vi "Setup.vi"(0 "Vector 26GHz Path Group in":refnum<class "Vector 26GHz Path Group.lvclass">, 11 "error in":errorcluster) -> (4 "Vector 26GHz Path Group out":refnum<class "Vector 26GHz Path Group.lvclass">, 15 "error out":errorcluster)   [LabVIEW 2023, in "RFFixtureCharact.RMM.lvlib" / "Vector 26GHz Path Group.lvclass"]
uses:
  Vector 26GHz Path Group.lvclass
  Vector 26GHz Path Group.lvclass/Vector 26GHz Path Group.ctl
  Paths/Vector Path/Vector 26GHz Path.lvclass
  Public/Base Classes/Vector/Vector Abstract Path/Vector Abstract Path.lvclass
  Common/RFCalAndFixtureCharact.Common.lvlib
  Public/Base Classes/Vector/Vector Path Group/Vector Path Group.lvclass
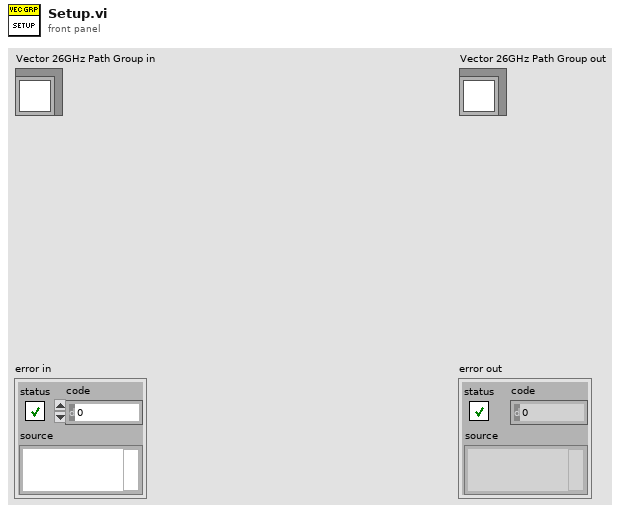
[diagram p1: front panel]
types:
  T1 = typedef "RFFixtureCharact.Public.lvlib/Vector Path Group.lvclass/Sweep.ctl" = cluster{"Port Power":dbl, "Frequencies":dbl[], "Test Receiver Attenuation":dbl, "IF Bandwidth":dbl}
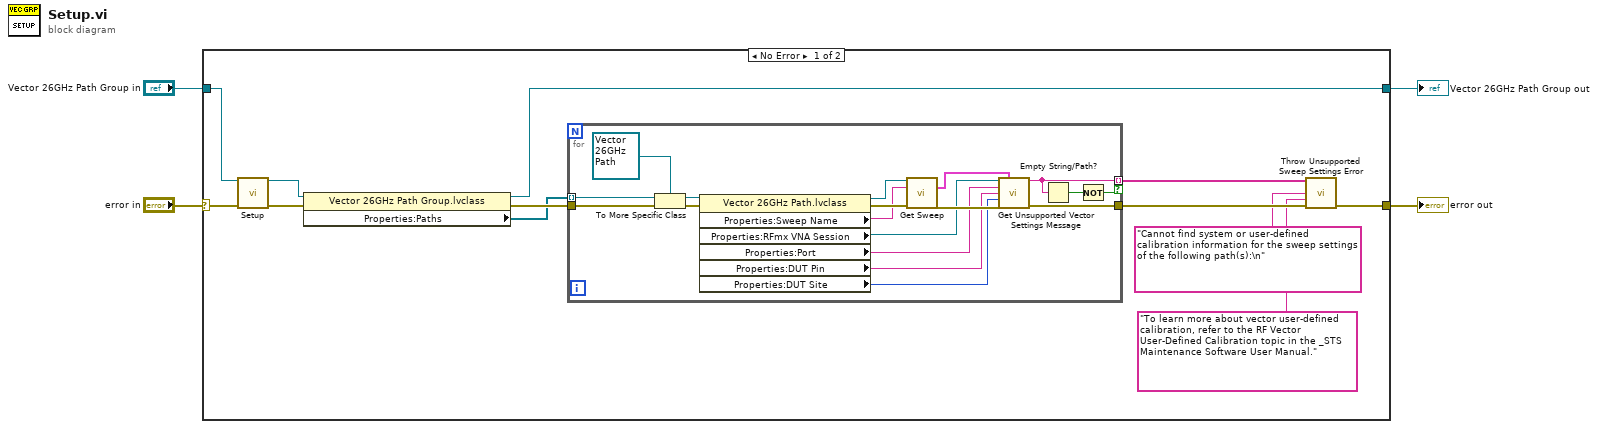
[diagram p0: block diagram]
diagram:
  n1 = case shown="No Error" "error in" {
    selector: "error in" -> [w16 w36]
    tunnel: [w14 w36] -> w2
    tunnel: [w9 w35] -> w1
    tunnel: "Vector 26GHz Path Group in" -> [w11 w35]
    frame No Error {
      n2 = call-parent "Setup.vi"("Path Group in"=w11, "error in"=w16) -> ("Path Group out"=w12:refnum<class "Vector 26GHz Path Group.lvclass">, "error out"=w13:errorcluster)  [unwired: 12 in]
      n3 = property class="Vector 26GHz Path Group.lvclass"(reference=w12, error in=w13) -> (reference out=w9:refnum<class "Vector 26GHz Path Group.lvclass">, error out=w10:errorcluster, "Properties:Paths"=w8:refnum<class "Path.lvclass">[])
      n4 = for {
        tunnel: w8 -> [w33] mode=indexing
        tunnel: w10 -> [w34]
        tunnel: [w24] -> w15
        tunnel: [w20] -> w7 mode=indexing if=w21
        n5 = To More Specific Class(target class=refnum<class "Vector 26GHz Path.lvclass"> refnum ("RFFixtureCharact.RMM.lvlib:Vector 26GHz Path.lvclass"), reference=w33, error in=w34) -> (specific class reference=w32:refnum<class "Vector 26GHz Path.lvclass">, error out=w31:errorcluster)
        n6 = property class="Vector 26GHz Path.lvclass"(reference=w32, error in=w31) -> (reference out=w18:refnum<class "Vector 26GHz Path.lvclass">, error out=w29:errorcluster, "Properties:Sweep Name"=w19:string, "Properties:RFmx VNA Session"=w27:refnum<k21>, "Properties:Port"=w26:string, "Properties:DUT Pin"=w25:string, "Properties:DUT Site"=w23:i32)
        n7 = call-dynamic "Get Sweep.vi"("Vector Path in"=w18, "Sweep Name"=w19, "error in (no error)"=w29) -> ("Sweep"=w17:T1, "error out"=w28:errorcluster)  [unwired: 9 in, 2 out]
        n8 = call "Get Unsupported Vector Settings Message.vi"("RFmx VNA Session"=w27, "Sweep"=w17, "Port"=w26, "DUT Pin"=w25, "DUT Site"=w23, "error in"=w28) -> ("Error Message"=w20:string, "error out"=w24:errorcluster)  [unwired: 8 in]
        n9 = Empty String/Path?(string/path=w20) -> (empty?=w22:bool)
        n10 = Not(x=w22) -> (.not. x?=w21:bool)
      }
      n11 = call "Throw Unsupported Sweep Settings Error.vi"("Error Message List"=w7, "Additional Header"="Cannot find system or user-defined calibration information for the sweep settings of the following path(s):\n" ("Error Message Header"), "Additional Details"="To learn more about vector user-defined calibration, refer to the RF Vector User-Defined Calibration topic in the _STS Maintenance Software User Manual.", "error in"=w15) -> ("error out"=w14:errorcluster)  [unwired: 11 in]
    }
    frame Error {
    }
  }
  "error out" <- w2
  "Vector 26GHz Path Group out" <- w1
